vi "Benchmark FIFO Read.vi"(6 "timed out?":bool, 8 "error in (no error)":errorcluster, 9 "T_Rx":i64, 10 "Header":T1, 11 "CIFCorePlugin in":refnum<class "CIFCorePlugin.lvclass">) -> (0 "error out":errorcluster, 3 "CIFCorePlugin out":refnum<class "CIFCorePlugin.lvclass">)   [LabVIEW 2021, in "CIFCorePlugin.lvclass"]
doc: "This will track the statistics for the fifo timing (how long was data in the channel fifo, both between this node and the last writer as well as from the initial time the data was created.)\n\nIt is automatically called in Channel reads in the class but should be manually for custom channels that were not added to the class data."
uses:
  CIFCorePlugin.lvclass
  <vilib>/CIF Foundation/CIF Channels Core/ChannelCommon/typedef/FIFO Header.ctl
  CIFCorePlugin.lvclass/CIFCorePlugin.ctl
  <vilib>/CIF Foundation/CIF Utilities/Statistics/I64/Stats_I64_CIF_U.lvclass/Stats_I64_CIF_U.ctl
  <vilib>/CIF Foundation/CIF Utilities/Statistics/I64/X1 minus X0.vi/dfabcf33-0dbc-4041-80a5-3dc0c86d2989.vi
  <vilib>/CIF Foundation/CIF Utilities/Time/System Time/LabVIEW Time to TAI Time.vi
  <vilib>/CIF Foundation/CIF Utilities/Statistics/I64/X1 minus X0.vi/dfabcf33-0dbc-4041-80a5-3dc0c86d2989.vi/9eb60a9a-770f-4d2d-8b3f-8465c267ecc9.vi
  <vilib>/CIF Foundation/CIF Utilities/Statistics/I64/Stats_I64_CIF_U.lvclass
  <vilib>/CIF Foundation/CIF Utilities/Time/Time_CIF_U.lvlib
  <vilib>/CIF Foundation/CIF Channels Core/ChannelCommon/ChannelCommon.lvlib
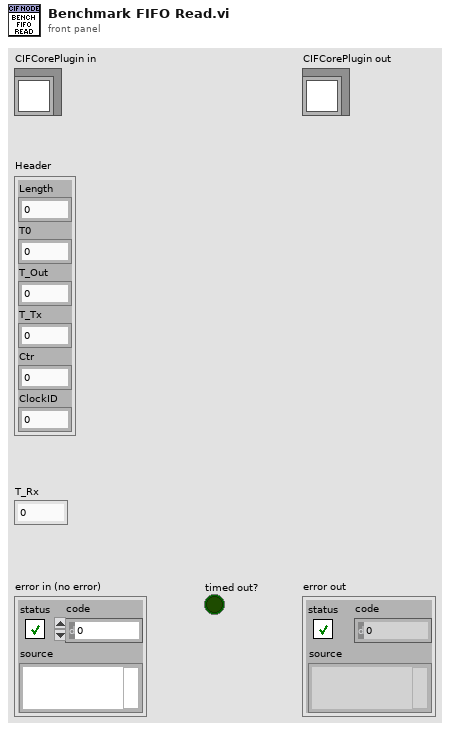
[diagram p1: front panel]
types:
  T1 = typedef "ChannelCommon.lvlib/FIFO Header.ctl" = cluster{"Length":u64, "T0":i64, "T_Out":i64, "T_Tx":i64, "Ctr":u64, "ClockID":u8}
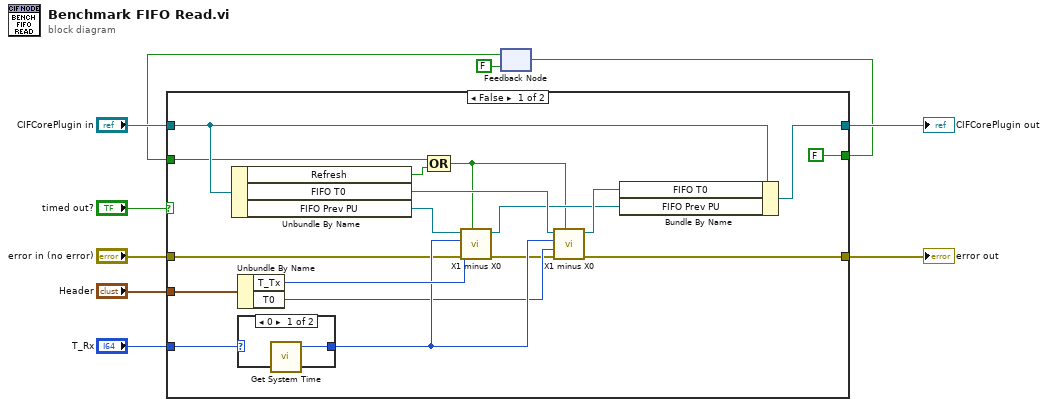
[diagram p0: block diagram]
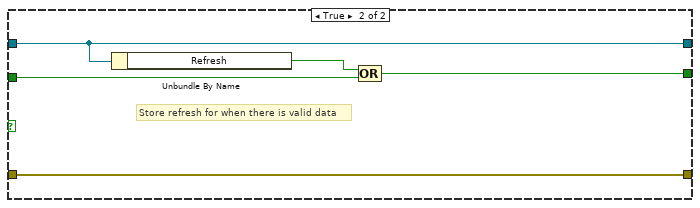
[diagram p3: hidden frame]
diagram:
  n1 = feedback #1(FALSE ("Refresh")) -> (w1:bool)
  n2 = case shown="False" "timed out?" {
    tunnel: [w16 w35] -> w10
    tunnel: [w26 w34] -> w8
    tunnel: "CIFCorePlugin in" -> [w27 w34]
    tunnel: "Header" -> [w25 _]
    tunnel: "T_Rx" -> [w23 _]
    tunnel: "error in (no error)" -> [w15 w35]
    tunnel: [FALSE w31] -> w2
    tunnel: w1 -> [w12 w32]
    frame False {
      n3 = Unbundle By Name(w27) -> ("Refresh"=w14:bool, "FIFO T0"=w22:refnum<class "Stats_I64_CIF_U.lvclass">, "FIFO Prev PU"=w28:refnum<class "Stats_I64_CIF_U.lvclass">)
      n4 = Unbundle By Name(w25) -> ("T_Tx"=w24:i64, "T0"=w20:i64)
      n5 = case shown="0" w23 {
        selector: w23 -> [_ w30]
        tunnel: [w29 w30] -> w21
        frame 0 {
          n6 = call <vilib>:"Get System Time.vi"() -> ("Time (ns)"=w29:i64)  [unwired: 5 in]
        }
        frame 1, Default {
        }
      }
      n7 = Compound Arithmetic op=OR(w12, w14) -> (w13:bool)
      n8 = call <vilib>:"X1 minus X0.vi"("Reinit"=w13, "error in (no error)"=w15, "X0"=w24, "X1"=w21, "Stats_I64_CIF_U in"=w28) -> ("error out"=w17:errorcluster, "Stats_I64_CIF_U out"=w18:refnum<class "Stats_I64_CIF_U.lvclass">)  [unwired: 5 in]
      n9 = call <vilib>:"X1 minus X0.vi"("Reinit"=w13, "error in (no error)"=w17, "X0"=w20, "X1"=w21, "Stats_I64_CIF_U in"=w22) -> ("error out"=w16:errorcluster, "Stats_I64_CIF_U out"=w19:refnum<class "Stats_I64_CIF_U.lvclass">)  [unwired: 5 in]
      n10 = Bundle By Name(cluster=w27, "FIFO T0"=w19, "FIFO Prev PU"=w18) -> (w26:refnum<class "CIFCorePlugin.lvclass">)
    }
    frame True {
      # "Store refresh for when there is valid data"
      n11 = Unbundle By Name(w34) -> ("Refresh"=w33:bool)
      n12 = Compound Arithmetic op=OR(w33, w32) -> (w31:bool)
    }
  }
  "error out" <- w10
  "CIFCorePlugin out" <- w8
  n13 = feedback-in #1(w2) -> ()
